vi "panStamp_beconRX.vi"() -> ()   [LabVIEW 2014]
uses:
  Program Files (x86)/National Instruments/LabVIEW 2014/examples/Instrument IO/Serial/support/Serial - Settings.ctl
  <vilib>/Instr/_visa.llb/VISA Configure Serial Port (Instr).vi
panel:
  in  "Clear":bool
  in  "Stop Button":bool
  out "lqi level":u8(slide) scale=0.0..64.0
  out "door 2":bool
  out "door 1":bool
  out "rssi level":dbl(slide)
  out "temp plot":dbl[](graph)
  out "rssi":dbl[](graph)
  out "?":T1
  in  "delay before read (ms)":u32=500
  out "Response":string
  in  "Serial Settings":T2={"baud rate"=9600, "data bits"=8, "parity"=enum."None", "stop bits"=10, "flow control"=0} {"flow control" items=["None"=0, "XON/XOFF"=1, "RTS/CTS"=2, "DTR/DSR"=4]; "stop bits" items=["1.0"=10, "1.5"=15, "2.0"=20]; "data bits" min=5 max=8 step=1; "baud rate" items=["75"=75, "110"=110, "134"=134, "150"=150, "300"=300, "600"=600, "1200"=1200, "1800"=1800, "2400"=2400, "4800"=4800, "7200"=7200, "9600"=9600, "14400"=14400, "19200"=19200, "28800"=28800, "38400"=38400, "56000"=56000, "57600"=57600, "115200"=115200, "128000"=128000, "230400"=230400]}
  in  "VISA resource name":refnum<visa-resource-name>
  # "dBm"
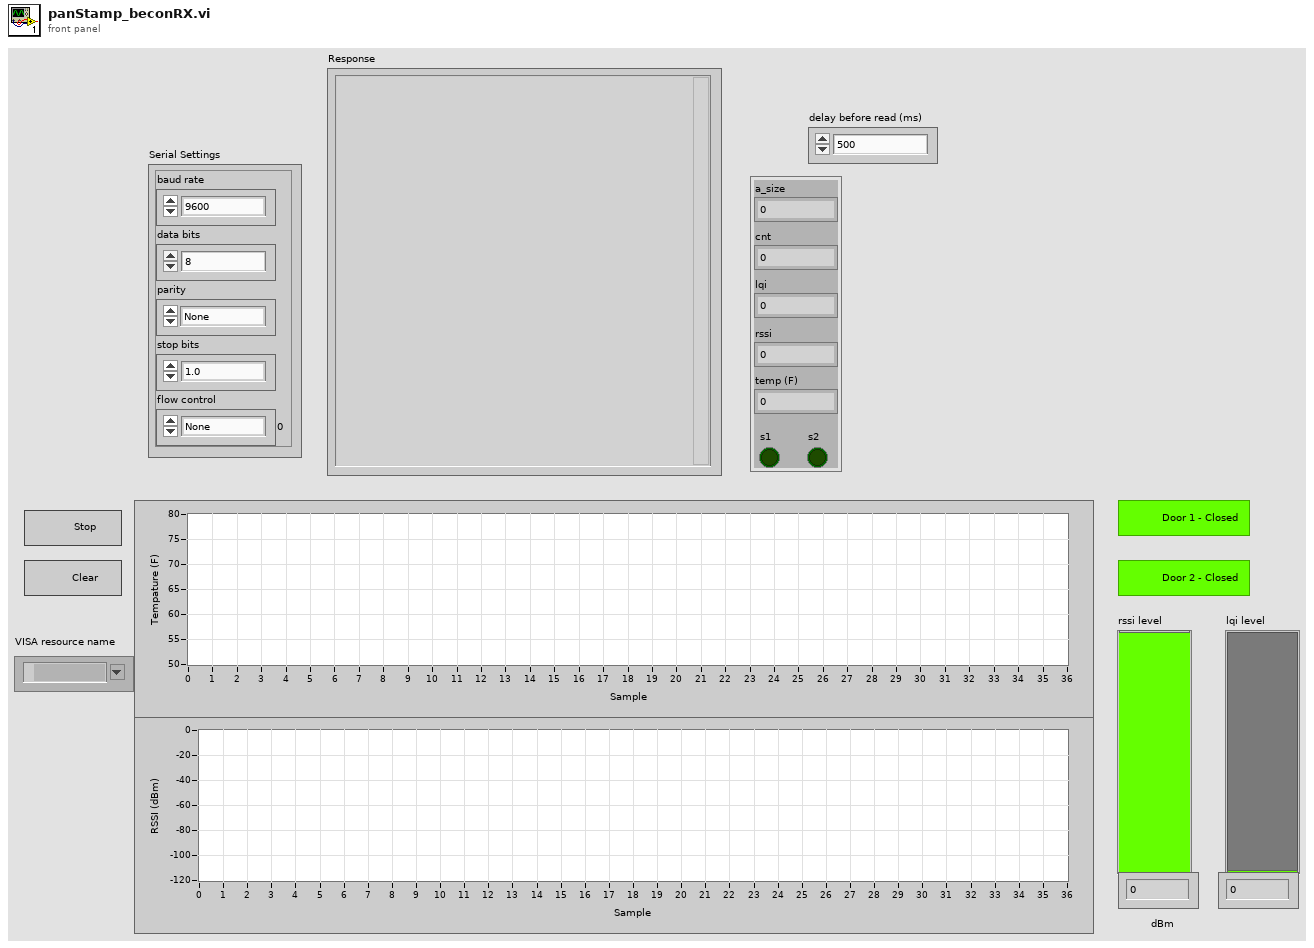
[diagram p1: front panel]
types:
  T1 = cluster{"rssi":dbl, "a_size":i32, "lqi":u8, "cnt":dbl, "s1":bool, "s2":bool, "temp (F)":dbl}
  T2 = typedef "Serial - Settings.ctl" = cluster{"baud rate":u32, "data bits":u16, "parity":enum16{"None", "Odd", "Even", "Mark", "Space"}, "stop bits":u16, "flow control":u16}
  T3 = cluster{"rssi":dbl, "a_size":i32, "lqi":u8, "cnt":dbl, "s1":bool, "s2":bool, "temp":dbl}
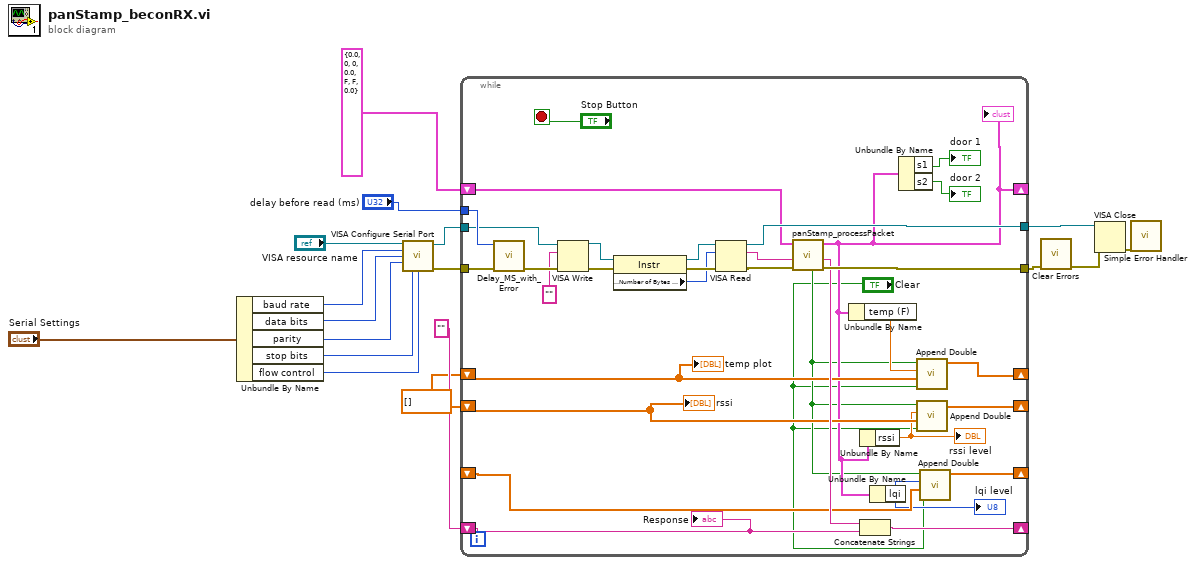
[diagram p0: block diagram]
diagram:
  w1 = dbl[] [] ("appended array")
  n1 = Unbundle By Name("Serial Settings") -> ("baud rate"=w15:u32, "data bits"=w14:u16, "parity"=w13:enum16{"None", "Odd", "Even", "Mark", "Space"}, "stop bits"=w12:u16, "flow control"=w11:u16)
  n2 = call-poly "VISA Configure Serial Port"("VISA resource name"="VISA resource name", "baud rate (9600)"=w15, "data bits (8)"=w14, "parity (0:none)"=w13, "stop bits (10: 1 bit)"=w12, "flow control (0:none)"=w11) -> ("VISA resource name out"=w8:refnum<visa-resource-name>, "error out"=w10:errorcluster)  [unwired: 8 in]
  n3 = while {
    tunnel: w10 -> [w48]
    tunnel: "delay before read (ms)" -> [w47]
    tunnel: w8 -> [w44]
    shift-right: [w26] -> _
    shift-left: "" -> [w25]
    tunnel: [w40] -> w6
    tunnel: [w39] -> w4
    shift-right: [w24] -> _
    shift-left: T3 {"rssi"=0.0, "a_size"=0, "lqi"=0, "cnt"=0.0, "s1"=FALSE, "s2"=FALSE, "temp"=0.0} -> [w36]
    shift-right: [w28] -> _
    shift-left: w1 -> [w29]
    shift-right: [w31] -> _
    shift-left: w1 -> [w32]
    shift-right: [w21] -> _
    shift-left: _ -> [w22]
    stop <- "Stop Button" stop-if-true
    n4 = call "Delay_MS_with_Error.vi"("error in"=w48, "delay before read (ms)"=w47) -> ("error out"=w45:errorcluster)  [unwired: 9 in]
    n5 = VISA Write(VISA resource name=w44, write buffer="", error in (no error)=w45) -> (VISA resource name out=w42:refnum<visa-resource-name>, error out=w46:errorcluster)  [unwired: 1 out]
    n6 = property class="Instr"(reference=w42, error in=w46) -> (reference out=w49:refnum<visa-resource-name>, error out=w50:errorcluster, "Serial Settings:Number of Bytes at Serial Port"=w41:u32)
    n7 = VISA Read(VISA resource name=w49, byte count=w41, error in (no error)=w50) -> (VISA resource name out=w40:refnum<visa-resource-name>, read buffer=w37:string, error out=w38:errorcluster)  [unwired: 1 out]
    n8 = call "panStamp_processPacket.vi"("error in"=w38, "packet_in"=w37, "Status In"=w36) -> ("error out"=w39:errorcluster, "formatted text out"=w35:string, "Status Out"=w24:T1, "update"=w23:bool)  [unwired: 4 in, 1 out]
    "?" <- w24
    n9 = Unbundle By Name(w24) -> ("temp (F)"=w30:dbl)
    n10 = Unbundle By Name(w24) -> ("rssi"=w27:dbl)
    "rssi level" <- w27
    n11 = Concatenate Strings(w35, w25) -> (w26:string)
    n12 = Unbundle By Name(w24) -> ("lqi"=w20:u8)
    "lqi level" <- w20
    n13 = Unbundle By Name(w24) -> ("s1"=→"door 1":bool, "s2"=→"door 2":bool)
    n14 = call "Append Double.vi"("clear"="Clear", "Input Array"=w29, "Input Vale"=w30, "Update"=w23) -> ("Output Array"=w28:dbl[])  [unwired: 7 in]
    n15 = call "Append Double.vi"("clear"="Clear", "Input Array"=w32, "Input Vale"=w27, "Update"=w23) -> ("Output Array"=w31:dbl[])  [unwired: 7 in]
    n16 = call "Append Double.vi"("clear"="Clear", "Input Array"=w22, "Input Vale"=w20, "Update"=w23) -> ("Output Array"=w21:dbl[])  [unwired: 7 in]
    "Response" <- w25
    "temp plot" <- w29
    "rssi" <- w32
  }
  n17 = call <vilib>:"Clear Errors.vi"("error in (no error)"=w4) -> ("error out"=w5:errorcluster)  [unwired: 5 in, 1 out]
  n18 = VISA Close(VISA resource name=w6, error in (no error)=w5) -> (error out=w7:errorcluster)
  n19 = call <vilib>:"Simple Error Handler.vi"("error in (no error)"=w7) -> ()  [unwired: 1 in, 8 out]
